vi "releasePressureTest.vi"(7 "LabVIEW Web Service Request":refnum<class "Web Request.lvclass">, 9 "targetPressure":dbl, 10 "maximumTolerance":dbl, 11 "minimumTolerance":dbl) -> (2 "current pr":dbl, 3 "maximumPressure":dbl format="%0.2f")   [LabVIEW 2015]
uses:
  <vilib>/wsapi/Web Request.lvclass
  Control test 1.ctl
  <vilib>/Waveform/WDTOps.llb/WDT Append Waveforms DBL.vi
panel:
  out "value":string
  out "target_pr":dbl
  in  "stop (F)":bool
  out "data":T1
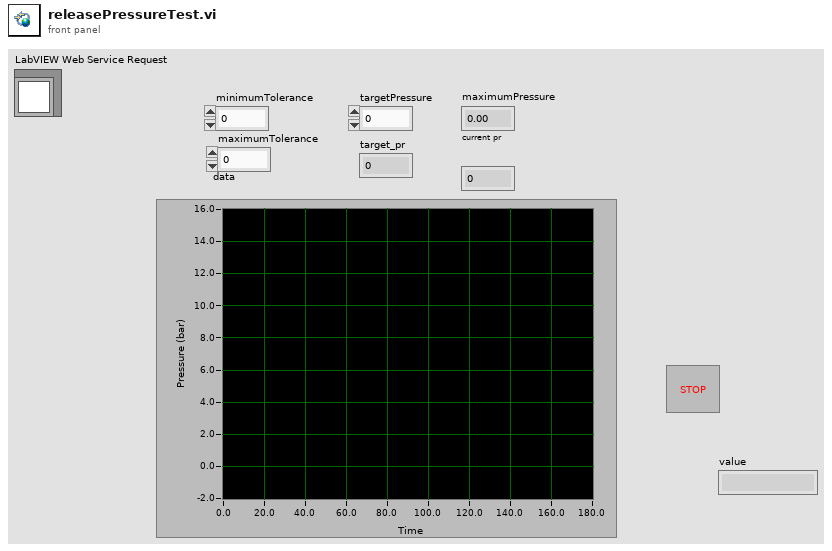
[diagram p1: front panel]
types:
  T1 = typedef "Control test 1.ctl" = dynamicdata
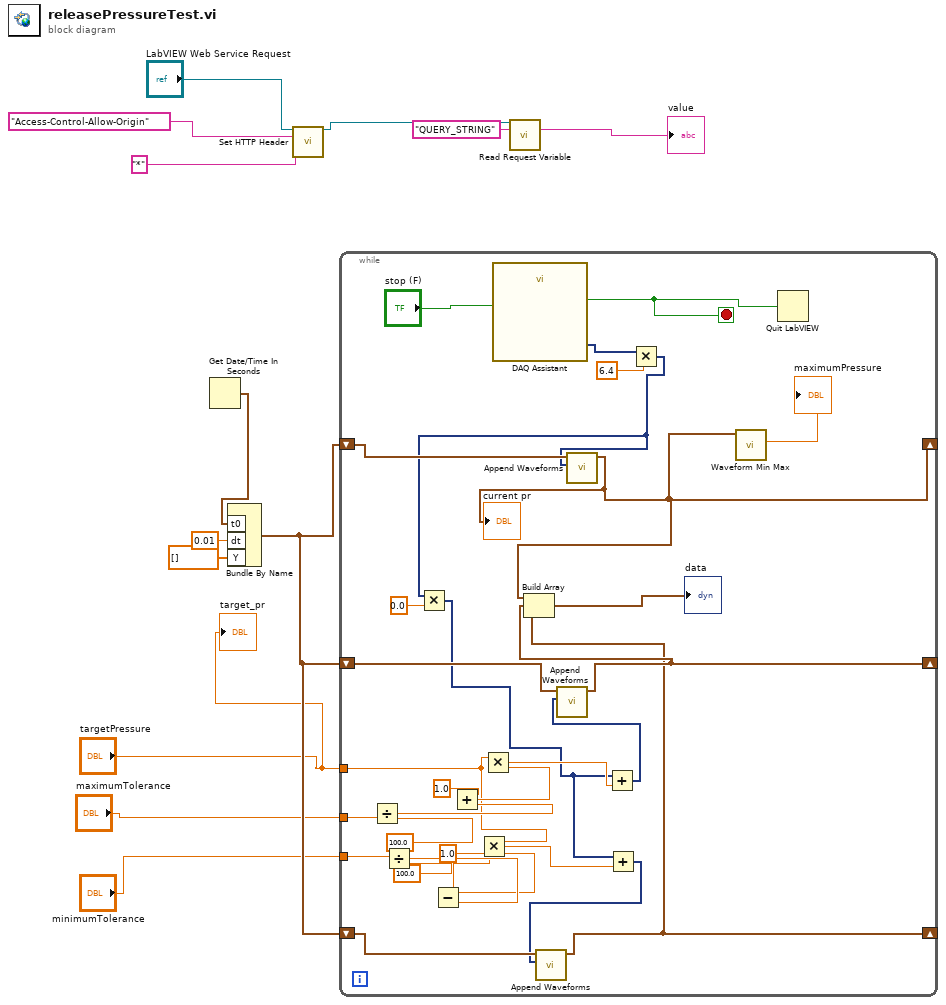
[diagram p0: block diagram]
diagram:
  n1 = Get Date/Time In Seconds() -> (seconds since 1Jan1904=w11:timestamp)
  n2 = Bundle By Name("t0"=w11, "dt"=0.01, "Y"=dbl[] []) -> (w10:waveform(dbl))  [unwired: 1 in]
  n3 = call <vilib>:"Set HTTP Header.vi"("LabVIEW Web Service Request"="LabVIEW Web Service Request", "header"="Access-Control-Allow-Origin", "header value"="*") -> ("LabVIEW Web Service Request out"=w3:refnum<class "Web Request.lvclass">)  [unwired: 11 in, 1 out]
  n4 = while {
    shift-right: [w16] -> _
    shift-left: w10 -> [w19]
    shift-right: [w40] -> _
    shift-left: w10 -> [w41]
    tunnel: "maximumTolerance" -> [w39]
    tunnel: "minimumTolerance" -> [w37]
    tunnel: "targetPressure" -> [w29]
    shift-right: [w24] -> _
    shift-left: w10 -> [w25]
    stop <- w14 stop-if-true
    n5 = Divide(x=w39, y=100.0) -> (x/y=w34:dbl)
    n6 = Divide(x=w37, y=100.0) -> (x/y=w33:dbl)
    n7 = Subtract(x=1.0, y=w33) -> (x-y=w31:dbl)
    n8 = Add(x=1.0, y=w34) -> (x+y=w30:dbl)
    n9 = Multiply(x=w29, y=w31) -> (x*y=w22:dbl)
    n10 = Multiply(x=w29, y=w30) -> (x*y=w27:dbl)
    n11 = call "DAQ Assistant"("stop (F)"="stop (F)") -> ("data"=w20:dynamicdata, "stopped"=w14:bool)  [unwired: 15 in, 2 out]
    n12 = Multiply(x=w20, y=6.4) -> (x*y=w17:dynamicdata)
    n13 = Multiply(x=w17, y=0.0) -> (x*y=w23:dynamicdata)
    n14 = call-poly <vilib>:"Append Waveforms.vi"("waveform B"=w17, "waveform A"=w19) -> ("waveform out"=w16:waveform(dbl))  [unwired: 8 in, 1 out]
    "current pr" <- w16
    n15 = Add(x=w23, y=w27) -> (x+y=w26:dynamicdata)
    n16 = call-poly <vilib>:"Append Waveforms.vi"("waveform B"=w26, "waveform A"=w41) -> ("waveform out"=w40:waveform(dbl))  [unwired: 8 in, 1 out]
    n17 = Add(x=w23, y=w22) -> (x+y=w21:dynamicdata)
    n18 = call-poly <vilib>:"Append Waveforms.vi"("waveform B"=w21, "waveform A"=w25) -> ("waveform out"=w24:waveform(dbl))  [unwired: 8 in, 1 out]
    n19 = Build Array(w16, w40, w24) -> (→"data":waveform(dbl)[])
    n20 = call <vilib>:"Waveform Min Max.vi"("waveform in"=w16) -> ("Y max"=→"maximumPressure":dbl)  [unwired: 5 in, 5 out]
    n21 = Quit LabVIEW(quit? (T)=w14) -> ()
  }
  n22 = call <vilib>:"Read Request Variable.vi"("LabVIEW Web Service Request"=w3, "variable name"="QUERY_STRING") -> ("value"=→"value":string)  [unwired: 11 in, 2 out]
  "target_pr" <- "targetPressure"
